vi "setUp.vi"(8 "error in (no error)":errorcluster, 11 "reference in":refnum<class "Bus Monitor Suite.lvclass">) -> (0 "error out":errorcluster, 3 "reference out":refnum<class "Bus Monitor Suite.lvclass">)   [LabVIEW 2016, in "Bus Monitor Suite.lvclass"]
doc: "setUp runs prior to the test method during test execution. Use this method to initialize any object data required by your tests."
uses:
  Bus Monitor Suite.lvclass
  <vilib>/addons/_JKI Toolkits/VI Tester/TestSuite.llb/TestSuite.lvclass
  Utilities/Simulated FPGA/FPGA Sim.lvclass
  1553 Test/1553 Test.lvclass
  D:/SVN/Products/BCI-1553/Software/Development/2016/RealTime/Utilities/FPGA Interface/FPGA Interface.lvclass
  PPLs/FPGA Interface.lvlibp/FPGA Interface/FPGA Interface.lvclass
  D:/Programs/National Instruments/LabVIEW 2016/vi.lib/addons/_JKI Toolkits/VI Tester/TestCase.llb/TestCase.lvclass
  D:/Programs/National Instruments/LabVIEW 2016/vi.lib/addons/_JKI Toolkits/VI Tester/TestSuite.llb/TestSuite.lvclass
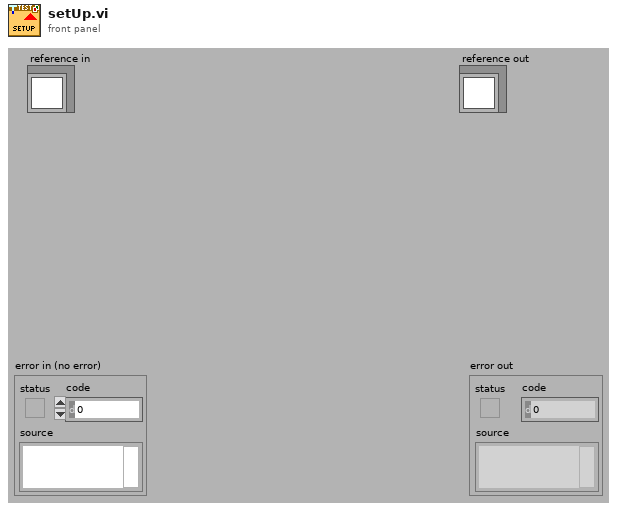
[diagram p1: front panel]
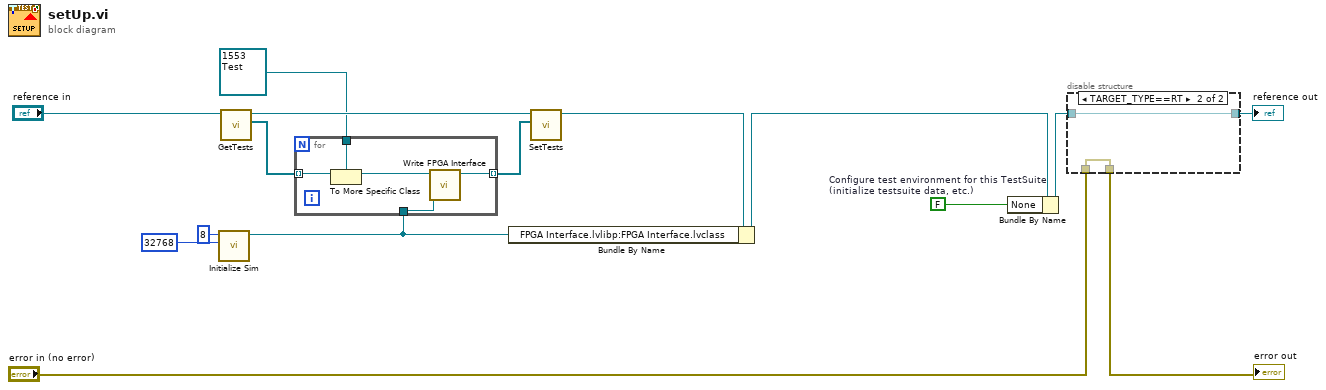
[diagram p0: block diagram]
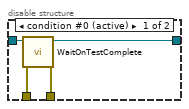
[diagram p2: hidden frame]
diagram:
  w15 = FALSE  # Configure test environment for this TestSuite  (initialize testsuite data, etc.)
  n1 = call "Initialize Sim.vi"("Memory Size (32k)"=32768, "Components (8)"=8) -> ("FPGA Sim out"=w3:refnum<class "FPGA Sim.lvclass">)  [unwired: 8 in, 1 out]
  n2 = call-dynamic "GetTests.vi"("TestSuite in"="reference in") -> ("tests"=w6:refnum<class>[], "TestSuite in"=w8:refnum<class "Bus Monitor Suite.lvclass">)  [unwired: 8 in, 1 out]
  n3 = for {
    tunnel: w6 -> [w20] mode=indexing
    tunnel: refnum<class "1553 Test.lvclass"> refnum ("1553 Test.lvclass") -> [w19]
    tunnel: [w17] -> w4 mode=indexing
    tunnel: w3 -> [w16]
    n4 = To More Specific Class(target class=w19, reference=w20) -> (specific class reference=w18:refnum<class "1553 Test.lvclass">)  [unwired: 1 in, 1 out]
    n5 = call-dynamic "Write FPGA Interface.vi"("FPGA Interface"=w16, "1553 Test in"=w18) -> ("1553 Test out"=w17:refnum<class "1553 Test.lvclass">)  [unwired: 8 in, 1 out]
  }
  n6 = call-dynamic "SetTests.vi"("tests"=w4, "TestSuite in"=w8) -> ("TestSuite in"=w7:refnum<class "Bus Monitor Suite.lvclass">)  [unwired: 8 in, 1 out]
  n7 = Bundle By Name(cluster=w7, "FPGA Interface.lvlibp:FPGA Interface.lvclass"=w3) -> (w1:refnum<class "Bus Monitor Suite.lvclass">)
  n8 = Bundle By Name(cluster=w1, "None"=w15) -> (w14:refnum<class "Bus Monitor Suite.lvclass">)
  n9 = disable-structure shown="TARGET_TYPE==RT" {
    disable-tunnel: w14 -> [w24 w25]
    disable-tunnel: [w23 w25] -> w13
    disable-tunnel: "error in (no error)" -> [w22 w26]
    disable-tunnel: [w21 w26] -> w11
    frame condition #0 (active) {
      n10 = call <vilib>:"WaitOnTestComplete.vi"("error in (no error)"=w22, "TestSuite in"=w24) -> ("error out"=w21:errorcluster, "TestSuite out"=w23:refnum<class "Bus Monitor Suite.lvclass">)  [unwired: 8 in]
    }
    frame condition #1 {
    }
  }
  "error out" <- w11
  "reference out" <- w13
